vi "Upload Configuration File.vi"(8 "error in (no error)":errorcluster, 10 "Config file to send":path, 11 "VISA resource name":refnum<visa-resource-name>) -> (0 "error out":errorcluster, 3 "VISA resource name out":refnum<visa-resource-name>)   [LabVIEW 2017, in "Sefram DAS220.lvlib"]
doc: "Upload a new configuration from your computer to the DAS240 as current configuration."
uses:
  <instrlib>/Sefram DAS220/Sefram DAS220.lvlib
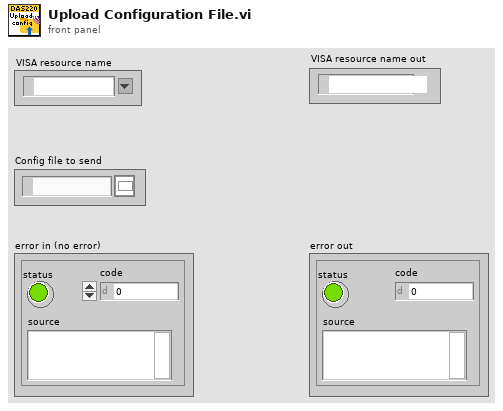
[diagram p1: front panel]
types:
  T1 = enum16{"big-endian, network order", "native, host order", "little-endian"}
  T2 = enum16{"open", "replace", "create", "open or create", "replace or create", "replace or create with confirmation"}
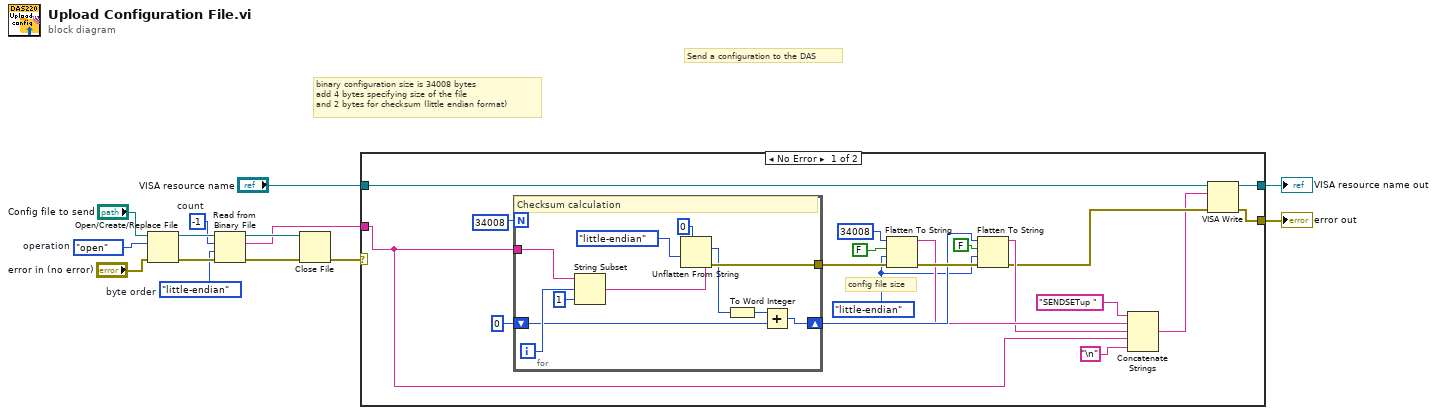
[diagram p0: block diagram]
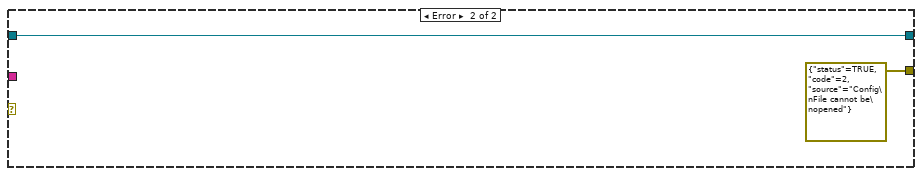
[diagram p2: hidden frame]
diagram:
  w7 = -1  # count
  w10 = T1."little-endian"  # byte order
  w14 = T2."open"  # operation
  # "binary configuration size is 34008 bytes\nadd 4 bytes specifying size of the file \nand 2 bytes for checksum (little endian format)"
  # "Send a configuration to the DAS"
  n1 = Open/Create/Replace File(file path (use dialog)="Config file to send", error in="error in (no error)", operation (0:open)=w14) -> (refnum out=w12:refnum<file>, error out=w11:errorcluster)  [unwired: 3 in, 1 out]
  n2 = Read from Binary File(8:w11, 9:w10, 10:w7, 11:w12) -> (0:w8:errorcluster, 2:w4:string, 3:w9:refnum<file>)  [unwired: 2 in, 1 out]
  n3 = Close File(refnum=w9, error in=w8) -> (error out=w6:errorcluster)  [unwired: 1 out]
  n4 = case shown="No Error" w6 {
    tunnel: w4 -> [w20 _]
    tunnel: "VISA resource name" -> [w25 w46]
    tunnel: [w18 w46] -> w2
    tunnel: [w17 errorcluster {"status"=TRUE, "code"=2, "source"="Config\nFile cannot be\nopened"} ("error constant")] -> w1
    frame No Error {
      w16 = T1."little-endian" ("byte order (0:big-endian, network order)")
      # "config file size"
      n5 = for {
        N: 34008 ("byte count") -> [_]
        tunnel: w20 -> [w44]
        tunnel: [w40] -> w31
        shift-right: [w37] -> w26
        shift-left: i16 0 -> [w38]
        i -> [w42]
        # "Checksum calculation"
        n6 = String Subset(string=w44, offset (0)=w42, length (rest)=1 ("length (rest)")) -> (substring=w39:string)
        n7 = Unflatten From String(type=u8 0, binary string=w39, byte order (0:big-endian, network order)=T1."little-endian") -> (value=w34:u8, error out=w40:errorcluster)  [unwired: 2 in, 1 out]
        n8 = To Word Integer(number=w34) -> (16bit integer=w35:i16)
        n9 = Add(x=w35, y=w38) -> (x+y=w37:i16)
      }
      n10 = Flatten To String(anything=34008, prepend array or string size? (T)=FALSE, byte order (0:big-endian, network order)=w16, error in (no error)=w31) -> (data string=w22:string, error out=w28:errorcluster)  [unwired: 1 out]
      n11 = Flatten To String(anything=w26, prepend array or string size? (T)=FALSE, byte order (0:big-endian, network order)=w16, error in (no error)=w28) -> (data string=w21:string, error out=w19:errorcluster)  [unwired: 1 out]
      n12 = Concatenate Strings("SENDSETup " ("string"), w22, w21, w20, "\n") -> (w15:string)
      n13 = VISA Write(VISA resource name=w25, write buffer=w15, error in (no error)=w19) -> (VISA resource name out=w18:refnum<visa-resource-name>, error out=w17:errorcluster)  [unwired: 1 out]
    }
    frame Error {
    }
  }
  "VISA resource name out" <- w2
  "error out" <- w1
